vi "System config bundler-DBL.vi"(7 "Keys setup.DBL":T5, 8 "error in (no error)":errorcluster, 9 "Section name":string, 10 "System Config I/P":T1={"Laser wavelength (nm)"=920.0, "DAQ FPGA System"={"Clock Freq (MHz) "=200.0, "Samples Wait after Trigger"=5080, "AOD fill"=4900, "StartupDelay"=0, "Slip Cycle (clock cycles)"=600000, "Add Cycle"=TRUE}, "Control system"={"AOD 1 Amplitude"=0, "AOD 2 Amplitude"=0, "AOD 3 Amplitude"=0, "AOD 4 Amplitude"=0, "AOD 5 Amplitude"=0, "AOD 6 Amplitude"=0, "T0 (ns)"=0.0, "Ta (ns)"=0.0, "Data Time Interval (ns)"=0.0, "Ctrl FPGA Clock (MHz)"=240.0}} {"Control system"."Ctrl FPGA Clock (MHz)" min=80.0 max=500.0 step=1.0; "Control system"."Data Time Interval (ns)" min=0.0 max=2048.0 step=1.0; "Control system"."Ta (ns)" min=0.0 max=2048.0 step=1.0; "Control system"."T0 (ns)" min=0.0 max=2048.0 step=1.0; "Control system"."AOD 6 Amplitude" min=0 max=2048 step=1; "Control system"."AOD 5 Amplitude" min=0 max=2048 step=1; "Control system"."AOD 4 Amplitude" min=0 max=2048 step=1; "Control system"."AOD 3 Amplitude" min=0 max=2048 step=1; "Control system"."AOD 2 Amplitude" min=0 max=2048 step=1; "Control system"."AOD 1 Amplitude" min=0 max=2048 step=1; "Laser wavelength (nm)" min=800.0 max=1080.0 step=1.0}, 11 "Refnum in":T4) -> (0 "error out":errorcluster, 2 "System Config O/P":T1={"Laser wavelength (nm)"=920.0, "DAQ FPGA System"={"Clock Freq (MHz) "=200.0, "Samples Wait after Trigger"=5080, "AOD fill"=4900, "StartupDelay"=0, "Slip Cycle (clock cycles)"=600000, "Add Cycle"=TRUE}, "Control system"={"AOD 1 Amplitude"=0, "AOD 2 Amplitude"=0, "AOD 3 Amplitude"=0, "AOD 4 Amplitude"=0, "AOD 5 Amplitude"=0, "AOD 6 Amplitude"=0, "T0 (ns)"=0.0, "Ta (ns)"=0.0, "Data Time Interval (ns)"=0.0, "Ctrl FPGA Clock (MHz)"=240.0}} {"Control system"."Ctrl FPGA Clock (MHz)" min=80.0 max=500.0 step=1.0; "Control system"."Data Time Interval (ns)" min=0.0 max=2048.0 step=1.0; "Control system"."Ta (ns)" min=0.0 max=2048.0 step=1.0; "Control system"."T0 (ns)" min=0.0 max=2048.0 step=1.0; "Control system"."AOD 6 Amplitude" min=0 max=2048 step=1; "Control system"."AOD 5 Amplitude" min=0 max=2048 step=1; "Control system"."AOD 4 Amplitude" min=0 max=2048 step=1; "Control system"."AOD 3 Amplitude" min=0 max=2048 step=1; "Control system"."AOD 2 Amplitude" min=0 max=2048 step=1; "Control system"."AOD 1 Amplitude" min=0 max=2048 step=1; "Laser wavelength (nm)" min=800.0 max=1080.0 step=1.0}, 3 "Refnum out":T4)   [LabVIEW 2017]
uses:
  Typedefs/Ini file interface (DBL).ctl
  <vilib>/Utility/config.llb/Config Data RefNum.ctl
  Typedefs/System Configuration.ctl
  Typedefs/DAQ FPGA system config.ctl
  Typedefs/CTRL system config.ctl
  <vilib>/Utility/config.llb/NI_LVConfig.lvlib
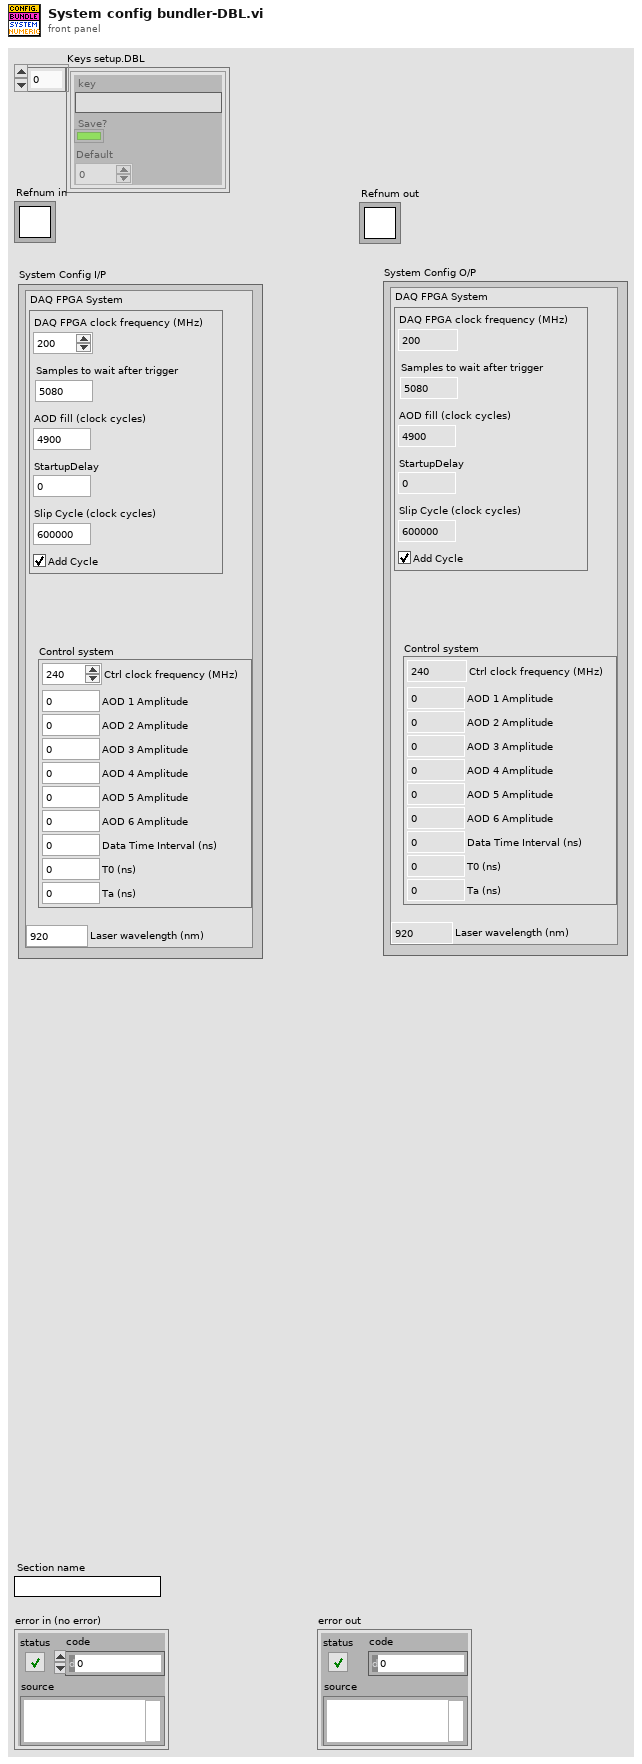
[diagram p1: front panel]
types:
  T1 = typedef "System Configuration.ctl" = cluster{"Laser wavelength (nm)":dbl, "DAQ FPGA System":T2, "Control system":T3}
  T2 = typedef "DAQ FPGA system config.ctl" = cluster{"Clock Freq (MHz) ":dbl, "Samples Wait after Trigger":u16, "AOD fill":u16, "StartupDelay":i32, "Slip Cycle (clock cycles)":u32, "Add Cycle":bool}
  T3 = typedef "CTRL system config.ctl" = cluster{"AOD 1 Amplitude":i16, "AOD 2 Amplitude":i16, "AOD 3 Amplitude":i16, "AOD 4 Amplitude":i16, "AOD 5 Amplitude":i16, "AOD 6 Amplitude":i16, "T0 (ns)":dbl, "Ta (ns)":dbl, "Data Time Interval (ns)":dbl, "Ctrl FPGA Clock (MHz)":dbl}
  T4 = typedef "NI_LVConfig.lvlib/Config Data RefNum.ctl" = refnum<k1>
  T5 = typedef "Ini file interface (DBL).ctl" = cluster{"key":string, "Save?":bool, "Default":dbl}[]
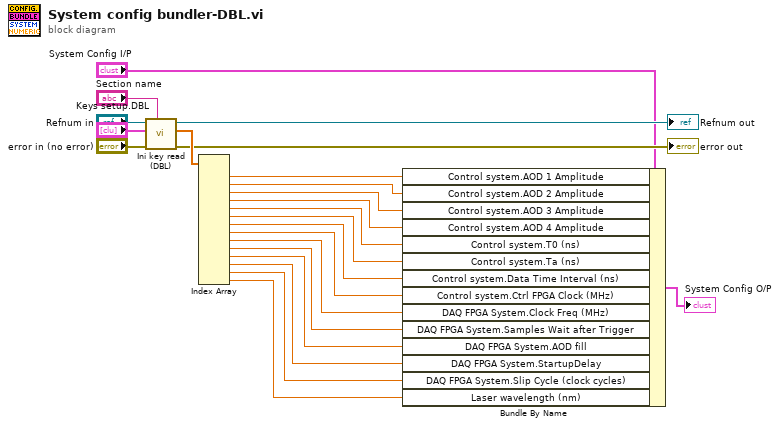
[diagram p0: block diagram]
diagram:
  n1 = call "Ini key read (DBL).vi"("Section name"="Section name", "error in (no error)"="error in (no error)", "Parameter names & setup"="Keys setup.DBL", "Ini file refnum in"="Refnum in") -> ("error out"=→"error out":errorcluster, "Value read/used"=w19:dbl[], "Ini file refnum out"=→"Refnum out":T4)  [unwired: 5 in]
  n2 = Index Array(array=w19) -> (element #1=w22:dbl, element #2=w23:dbl, element #3=w12:dbl, element #4=w11:dbl, element #5=w10:dbl, element #6=w9:dbl, element #7=w8:dbl, element #8=w7:dbl, element #9=w6:dbl, element #10=w5:dbl, element #11=w4:dbl, element #12=w3:dbl, element #13=w2:dbl, element #14=w1:dbl)  [unwired: 14 in]
  n3 = Bundle By Name(cluster="System Config I/P", "Control system.AOD 1 Amplitude"=w22, "Control system.AOD 2 Amplitude"=w23, "Control system.AOD 3 Amplitude"=w12, "Control system.AOD 4 Amplitude"=w11, "Control system.T0 (ns)"=w10, "Control system.Ta (ns)"=w9, "Control system.Data Time Interval (ns)"=w8, "Control system.Ctrl FPGA Clock (MHz)"=w7, "DAQ FPGA System.Clock Freq (MHz)"=w6, "DAQ FPGA System.Samples Wait after Trigger"=w5, "DAQ FPGA System.AOD fill"=w4, "DAQ FPGA System.StartupDelay"=w3, "DAQ FPGA System.Slip Cycle (clock cycles)"=w2, "Laser wavelength (nm)"=w1) -> (→"System Config O/P":T1)
